vi "Concatenate result strings.vi"(8 "Message":string, 9 "Description":string, 10 "Status":T1=enum."Passed", 11 "Input String":string) -> (3 "Output String":string)   [LabVIEW 2020, in "LUnit Test Case V2.lvclass"]
uses:
  LUnit Test Case V2.lvclass
  Result/Status.ctl
  LUnit Test Case V2.lvclass/LUnit Test Case V2.ctl
  Result/Result.lvlib
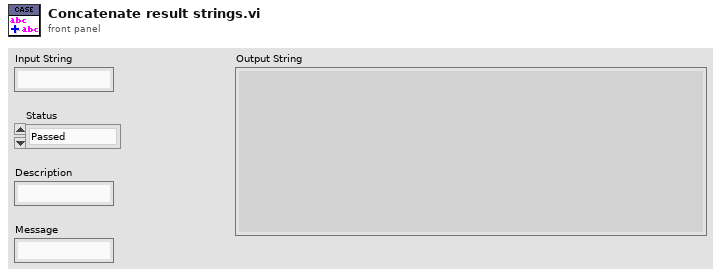
[diagram p1: front panel]
types:
  T1 = typedef "Result.lvlib/Status.ctl" = enum16{"", "Passed", "Failed", "Error", "Skipped", "Setup Error", "Broken", "Teardown Error"}
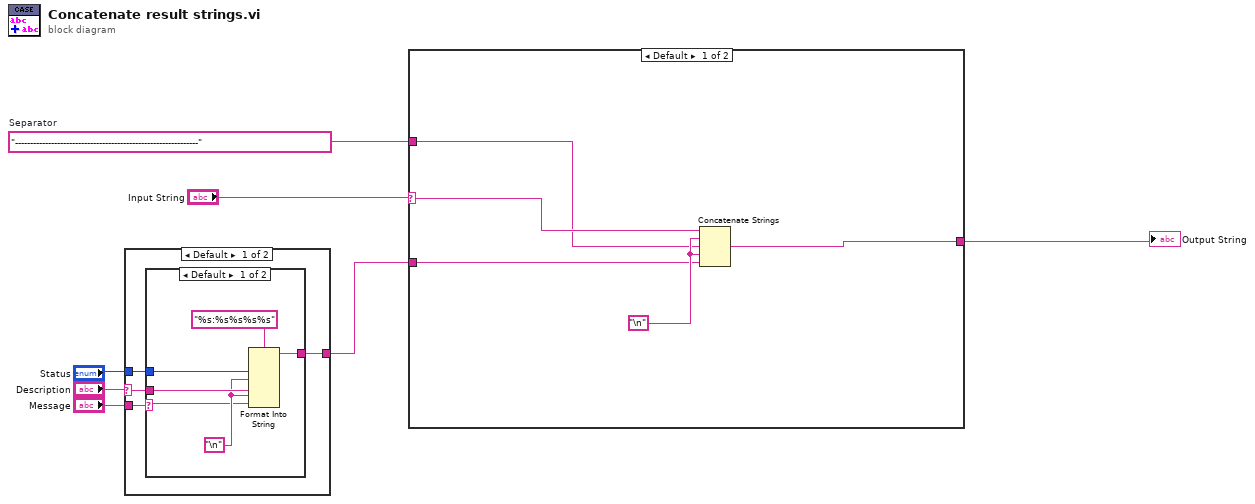
[diagram p0: block diagram]
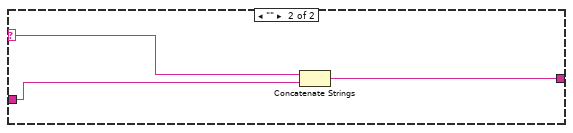
[diagram p2: hidden frame]
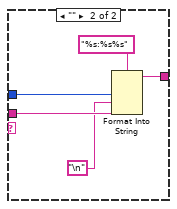
[diagram p3: hidden frame]
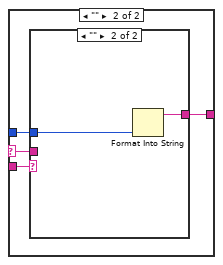
[diagram p4: hidden frame]
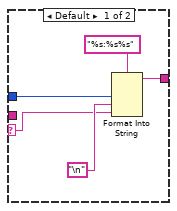
[diagram p5: hidden frame]
diagram:
  w7 = "-------------------------------------------------------------"  # Separator
  n1 = case shown="Default" "Description" {
    selector: "Description" -> [w10 w25]
    tunnel: "Status" -> [w11 w26]
    tunnel: "Message" -> [w9 w24]
    tunnel: [w8 w23] -> w2
    frame Default {
      n2 = case shown="Default" w9 {
        selector: w9 -> [w14 _]
        tunnel: w11 -> [w17 w21]
        tunnel: w10 -> [w16 w20]
        tunnel: [w13 w18] -> w8
        frame Default {
          w15 = "\n"
          n3 = Format Into String(format string="%s:%s%s%s%s", w17, w15, w16, w15, w14) -> (resulting string=w13:string)  [unwired: 2 in, 1 out]
        }
        frame "" {
          n4 = Format Into String(format string="%s:%s%s", w21, "\n", w20) -> (resulting string=w18:string)  [unwired: 2 in, 1 out]
        }
      }
    }
    frame "" {
      n5 = case shown="\"\"" w24 {
        selector: w24 -> [w29 _]
        tunnel: w26 -> [w31 w33]
        tunnel: w25 -> [_ _]
        tunnel: [w28 w32] -> w23
        frame Default {
          n6 = Format Into String(format string="%s:%s%s", w31, "\n", w29) -> (resulting string=w28:string)  [unwired: 2 in, 1 out]
        }
        frame "" {
          n7 = Format Into String(w33) -> (resulting string=w32:string)  [unwired: 3 in, 1 out]
        }
      }
    }
  }
  n8 = case shown="Default" "Input String" {
    selector: "Input String" -> [w37 w39]
    tunnel: w2 -> [w35 w41]
    tunnel: w7 -> [w34 _]
    tunnel: [w38 w40] -> w1
    frame Default {
      w36 = "\n"
      n9 = Concatenate Strings(w37, w36, w34, w36, w35) -> (w38:string)
    }
    frame "" {
      n10 = Concatenate Strings(w39, w41) -> (w40:string)
    }
  }
  "Output String" <- w1
